vi "getScreenViPath.vi"(7 "Enum Screen":T1, 8 "error in (no error)":errorcluster) -> (0 "error out":errorcluster, 3 "Path":path)   [LabVIEW 2013]
uses:
  enumScreen.ctl
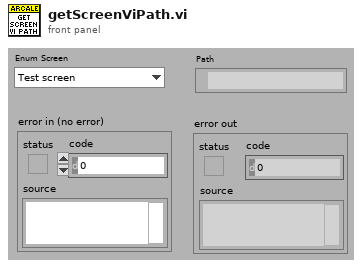
[diagram p1: front panel]
types:
  T1 = typedef "enumScreen.ctl" = enum16{"Test screen", "Ecran principal", "LOG", "Setup", "Popup : About", "Popup : View last message", "Popup : WebBrowser help", "Traduction", "Popup : DEBUG Process"}
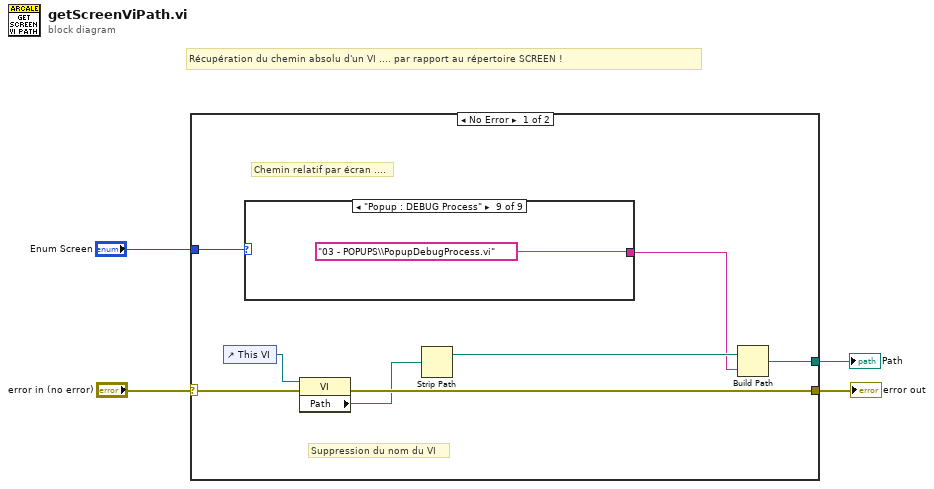
[diagram p0: block diagram]
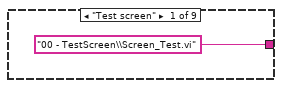
[diagram p2: hidden frame]
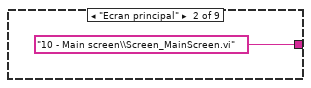
[diagram p3: hidden frame]
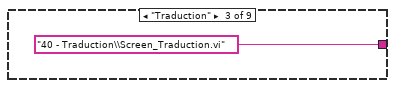
[diagram p4: hidden frame]
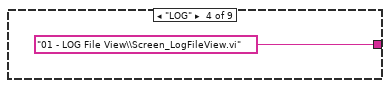
[diagram p5: hidden frame]
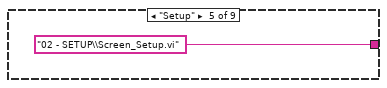
[diagram p6: hidden frame]
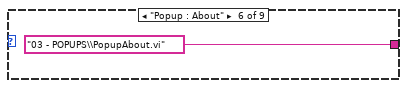
[diagram p7: hidden frame]
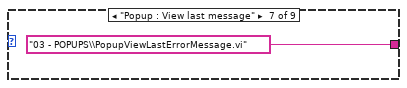
[diagram p8: hidden frame]
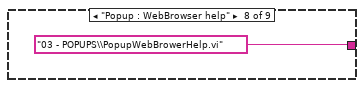
[diagram p9: hidden frame]
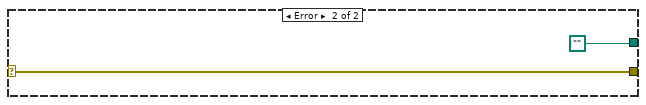
[diagram p10: hidden frame]
diagram:
  # "Récupération du chemin absolu d'un VI .... par rapport au répertoire SCREEN !"
  n1 = case shown="No Error" "error in (no error)" {
    selector: "error in (no error)" -> [w10 w23]
    tunnel: [w12 w23] -> w4
    tunnel: "Enum Screen" -> [w8 _]
    tunnel: [w5 path ""] -> w1
    frame No Error {
      # "Chemin relatif par écran ...."
      # "Suppression du nom du VI"
      n2 = control-ref of="This VI"() -> (w11:refnum<vi>)
      n3 = case shown="\"Popup : DEBUG Process\"" w8 {
        tunnel: ["00 - TestScreen\\Screen_Test.vi" "10 - Main screen\\Screen_MainScreen.vi" "40 - Traduction\\Screen_Traduction.vi" "01 - LOG File View\\Screen_LogFileView.vi" "02 - SETUP\\Screen_Setup.vi" "03 - POPUPS\\PopupAbout.vi" "03 - POPUPS\\PopupViewLastErrorMessage.vi" "03 - POPUPS\\PopupWebBrowerHelp.vi" "03 - POPUPS\\PopupDebugProcess.vi"] -> w6
        frame "Test screen" {
        }
        frame "Ecran principal" {
        }
        frame "Traduction" {
        }
        frame "LOG" {
        }
        frame "Setup" {
        }
        frame "Popup : About" {
        }
        frame "Popup : View last message" {
        }
        frame "Popup : WebBrowser help" {
        }
        frame "Popup : DEBUG Process" {
        }
      }
      n4 = property class="VI"(reference=w11, error in=w10) -> (error out=w12:errorcluster, "Path"=w9:path)  [unwired: 1 out]
      n5 = Strip Path(path=w9) -> (stripped path=w7:path)  [unwired: 1 out]
      n6 = Build Path(base path=w7, name or relative path=w6) -> (appended path=w5:path)
    }
    frame Error {
    }
  }
  "error out" <- w4
  "Path" <- w1
